vi "timer.vi"(10 "Elapsed Time (s)":dbl, 11 "string":string) -> (3 "String":string)   [LabVIEW 2015]
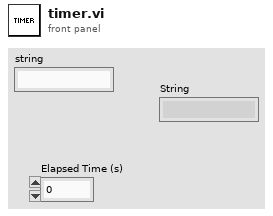
[diagram p1: front panel]
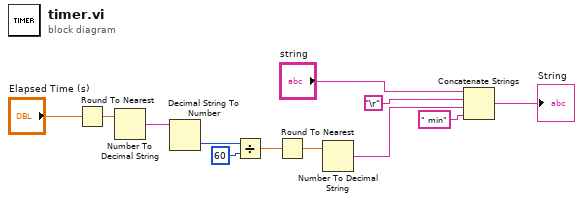
[diagram p0: block diagram]
diagram:
  n1 = Round To Nearest(number="Elapsed Time (s)") -> (nearest integer value=w3:dbl)
  n2 = Number To Decimal String(number=w3) -> (decimal integer string=w7:string)  [unwired: 1 in]
  n3 = Decimal String To Number(string=w7) -> (number=w8:i32)  [unwired: 2 in, 1 out]
  n4 = Divide(x=w8, y=60) -> (x/y=w10:dbl)
  n5 = Round To Nearest(number=w10) -> (nearest integer value=w11:dbl)
  n6 = Number To Decimal String(number=w11) -> (decimal integer string=w12:string)  [unwired: 1 in]
  n7 = Concatenate Strings("string", "\r", w12, " min" ("string")) -> (→"String":string)
